vi "FPGA_DIOWriteFilterPeriod.vi"(6 "DIOChannel":T1, 8 "error in (no error)":errorcluster, 9 "PWMFilterPeriod":u32, 10 "filter index":u8, 11 "DIODeviceRef In":T2) -> (0 "error out":errorcluster, 3 "DIODeviceRef Out":T2)   [LabVIEW 2017]
uses:
  <vilib>/Rock Robotics/SystemInterfaces/DIO/FPGA_DIODevRef.ctl
  <vilib>/Rock Robotics/SystemInterfaces/DIO/FPGA_DIOChannel.ctl
  <vilib>/Rock Robotics/SystemInterfaces/System/FPGA_SystemFPGA Ref Global.vi
  <vilib>/Utility/error.llb/Error Cluster From Error Code.vi
  <vilib>/rvi/errors/niLvFpgaAdjustHostInterfaceError.vi
  <vilib>/rvi/interface/nirviReadWriteControl/nirviReadWriteControl.xnode
  <vilib>/Rock Robotics/SystemInterfaces/System/FPGA_SystemFRC FPGA Ref.ctl
  NiFpgaLv.dll
  <vilib>/rvi/interface/Simulation/niFpgaSimulationCallBeginRW.vi
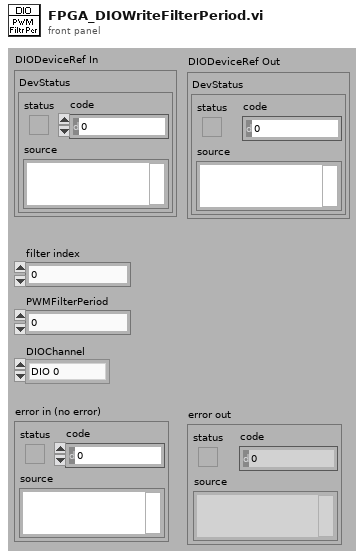
[diagram p1: front panel]
types:
  T1 = typedef "FPGA_DIOChannel.ctl" = enum8{"DIO 0", "DIO 1", "DIO 2", "DIO 3", "DIO 4", "DIO 5", "DIO 6", "DIO 7", "DIO 8", "DIO 9", "DIO MXP 0", "DIO MXP 1", "DIO MXP 2", "DIO MXP 3", "DIO MXP 4", "DIO MXP 5", "DIO MXP 6", "DIO MXP 7", "DIO MXP 8", "DIO MXP 9", "DIO MXP 10", "DIO MXP 11", "DIO MXP 12", "DIO MXP 13", "DIO MXP 14", "DIO MXP 15", "SPI Port CS1", "SPI Port CS2", "SPI Port CS3", "SPI Port MISO", "SPI Port MOSI", "Invalid"}
  T2 = typedef "FPGA_DIODevRef.ctl" = cluster{"DevStatus":errorcluster}
  T3 = typedef "FPGA_SystemFRC FPGA Ref.ctl" = refnum<k20>
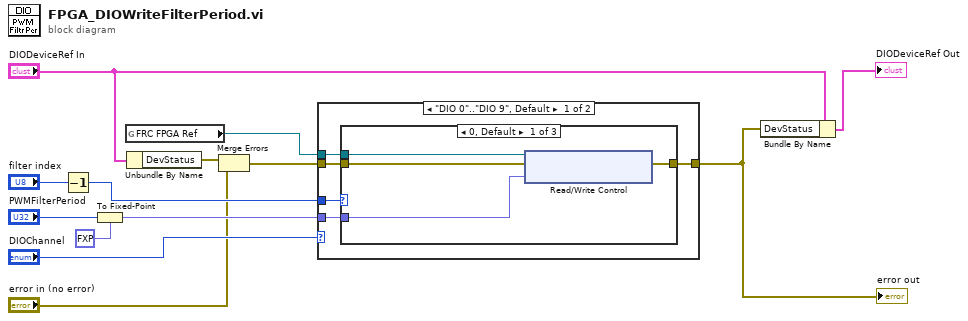
[diagram p0: block diagram]
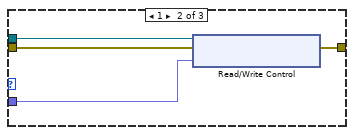
[diagram p2: hidden frame]
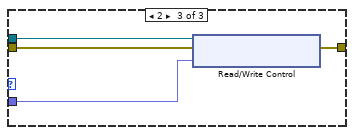
[diagram p3: hidden frame]
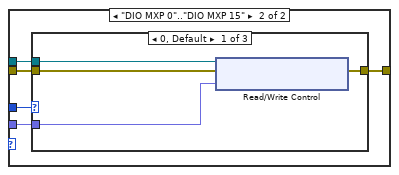
[diagram p4: hidden frame]
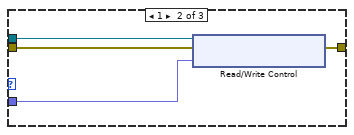
[diagram p5: hidden frame]
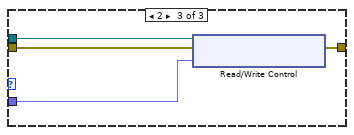
[diagram p6: hidden frame]
diagram:
  n1 = Decrement(x="filter index") -> (x-1=w4:u8)
  n2 = To Fixed-Point(fixed-point type=fxp<+,24,24> 0.0 ("DIO.FilterPeriodHdr0"), number="PWMFilterPeriod") -> (fixed-point=w3:fxp<+,24,24>)
  n3 = global read "FPGA_SystemFPGA Ref Global.vi" "FRC FPGA Ref"() -> (w7:T3)
  n4 = Unbundle By Name("DIODeviceRef In") -> ("DevStatus"=w9:errorcluster)
  n5 = Merge Errors(w9, "error in (no error)") -> (w8:errorcluster)
  n6 = case shown="\"DIO 0\"..\"DIO 9\", Default" "DIOChannel" {
    tunnel: [w18 w35] -> w6
    tunnel: w3 -> [w17 w34]
    tunnel: w4 -> [w14 w31]
    tunnel: w7 -> [w16 w33]
    tunnel: w8 -> [w15 w32]
    frame "DIO 0".."DIO 9", Default {
      n7 = case shown="0, Default" w14 {
        tunnel: [w22 w26 w30] -> w18
        tunnel: w17 -> [w21 w25 w29]
        tunnel: w16 -> [w20 w24 w28]
        tunnel: w15 -> [w19 w23 w27]
        frame 0, Default {
          n8 = xnode "Read/Write Control"("FPGA VI Reference In"=w20, "error in"=w19, "DIO.FilterPeriodHdr0"=w21) -> ("error out"=w22:errorcluster)  [unwired: 1 out]
        }
        frame 1 {
          n9 = xnode "Read/Write Control"("FPGA VI Reference In"=w24, "error in"=w23, "DIO.FilterPeriodHdr1"=w25) -> ("error out"=w26:errorcluster)  [unwired: 1 out]
        }
        frame 2 {
          n10 = xnode "Read/Write Control"("FPGA VI Reference In"=w28, "error in"=w27, "DIO.FilterPeriodHdr2"=w29) -> ("error out"=w30:errorcluster)  [unwired: 1 out]
        }
      }
    }
    frame "DIO MXP 0".."DIO MXP 15" {
      n11 = case shown="0, Default" w31 {
        tunnel: [w39 w43 w47] -> w35
        tunnel: w34 -> [w38 w42 w46]
        tunnel: w33 -> [w37 w41 w45]
        tunnel: w32 -> [w36 w40 w44]
        frame 0, Default {
          n12 = xnode "Read/Write Control"("FPGA VI Reference In"=w37, "error in"=w36, "DIO.FilterPeriodMXP0"=w38) -> ("error out"=w39:errorcluster)  [unwired: 1 out]
        }
        frame 1 {
          n13 = xnode "Read/Write Control"("FPGA VI Reference In"=w41, "error in"=w40, "DIO.FilterPeriodMXP1"=w42) -> ("error out"=w43:errorcluster)  [unwired: 1 out]
        }
        frame 2 {
          n14 = xnode "Read/Write Control"("FPGA VI Reference In"=w45, "error in"=w44, "DIO.FilterPeriodMXP2"=w46) -> ("error out"=w47:errorcluster)  [unwired: 1 out]
        }
      }
    }
  }
  "error out" <- w6
  n15 = Bundle By Name(cluster="DIODeviceRef In", "DevStatus"=w6) -> (→"DIODeviceRef Out":T2)
